vi "Inst_DAQ.vi"(8 "error in":errorcluster, 10 "All Message Queues in":T2, 11 "Prueba31 in":refnum<class "Prueba31.lvclass">) -> (0 "error out":errorcluster)   [LabVIEW 2019, in "Prueba31.lvclass"]
uses:
  Prueba31.lvclass
  QMH/Message Queue/All Message Queues.ctl
  QMH/Message Queue/Message Cluster.ctl
  Prueba31.lvclass/Prueba31.ctl
  <vilib>/DAQmx/write.llb/DAQmx Write (Analog 1D Wfm NChan NSamp).vi
  <vilib>/DAQmx/read.llb/DAQmx Read (Analog Wfm 1Chan 1Samp).vi
  <vilib>/Utility/error.llb/Error Cluster From Error Code.vi
  QMH/Message Queue/Enqueue Message (Single).vi
  <vilib>/DAQmx/create/channels.llb/DAQmx Create Channel (AO-Voltage-Basic).vi
  <vilib>/DAQmx/configure/timing.llb/DAQmx Timing (Sample Clock).vi
  <vilib>/DAQmx/miscellaneous.llb/DAQmx Fill In Error Info.vi
  <vilib>/DAQmx/create/channels.llb/DAQmx Create Channel (AI-Voltage-Basic).vi
  <vilib>/measure/matone.llb/Harmonic Distortion Analyzer 1 Chan.vi
  <vilib>/ErrorRing/Error Ring.xnode
  QMH/Message Queue/Message Queue.lvlib
  Instrumento/CNT90/CNT90.lvclass
  <vilib>/measure/NI_MAPro.lvlib
  <vilib>/measure/NI_MABase.lvlib
panel:
  in  "Output Array":T1(array[cluster])=[{"Waveform Type"=0, "Amplitude"=1.0, "Frequency"=10.0}] {"Frequency" format="%0.2p"; "Amplitude" format="%0.2p"; "Waveform Type" items=["Sine Wave", "Triangle Wave", "Square Wave", "Sawtooth Wave"]}
  out "All States":string[](array[string])
  out "Actual State":string
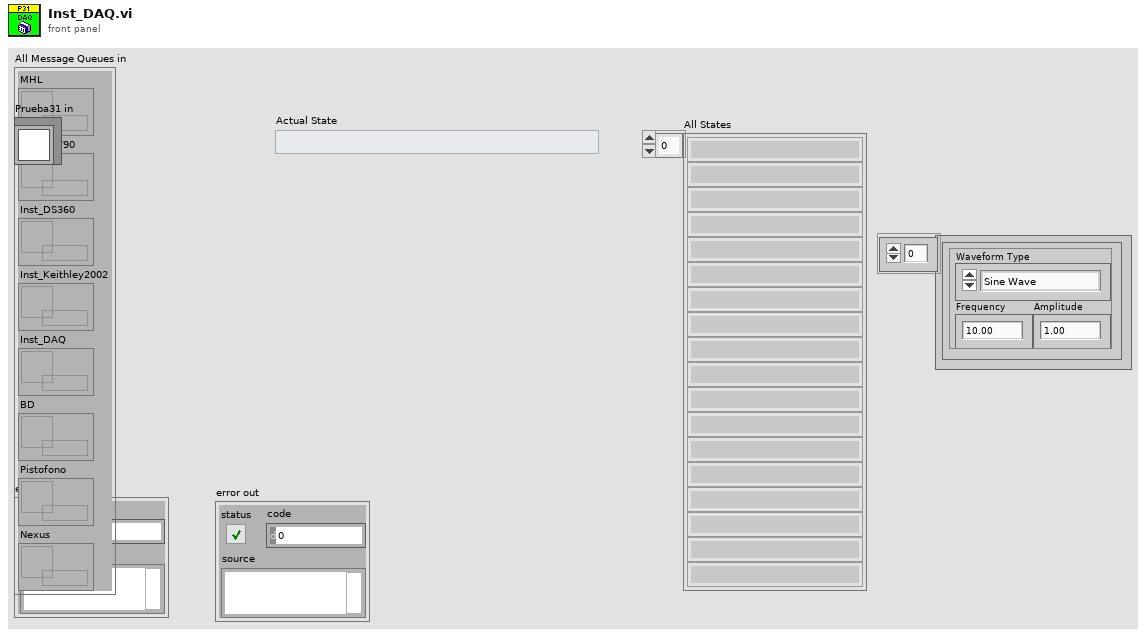
[diagram p1: front panel]
types:
  T1 = cluster{"Waveform Type":u16, "Amplitude":dbl, "Frequency":dbl}[]
  T2 = typedef "Message Queue.lvlib/All Message Queues.ctl" = cluster{"MHL":refnum<queue>, "Inst_CNT90":refnum<queue>, "Inst_DS360":refnum<queue>, "Inst_Keithley2002":refnum<queue>, "Inst_DAQ":refnum<queue>, "BD":refnum<queue>, "Pistofono":refnum<queue>, "Nexus":refnum<queue>}
  T3 = cluster{"Waveform Type":u16, "Amplitude":dbl, "Frequency":dbl}
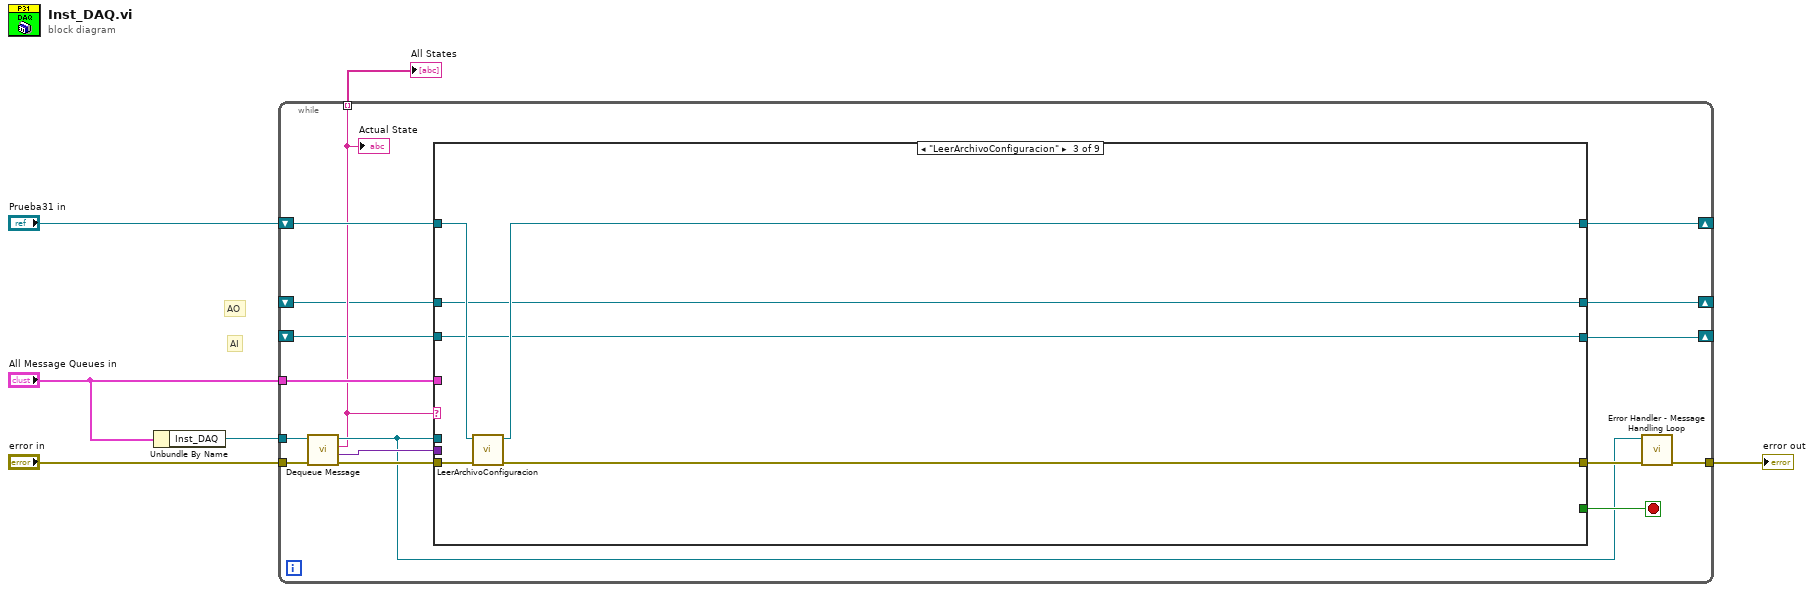
[diagram p0: block diagram]
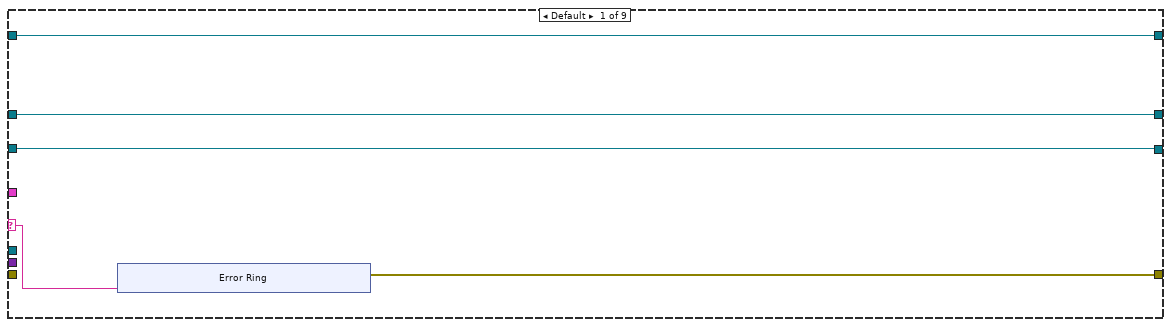
[diagram p2: hidden frame]
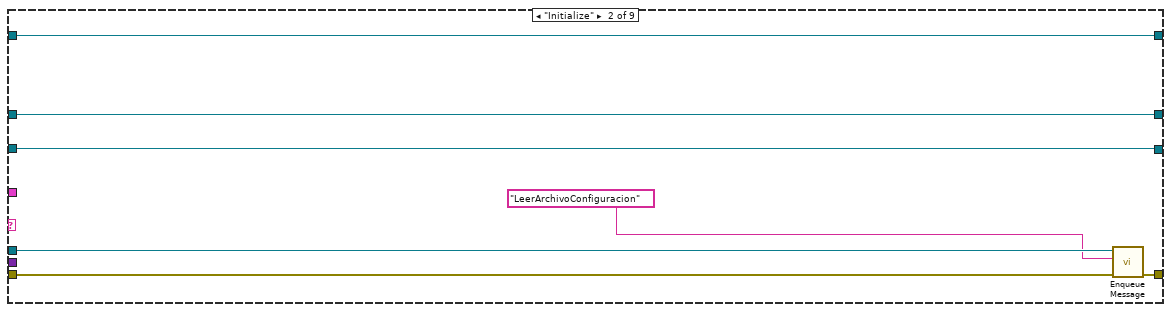
[diagram p3: hidden frame]
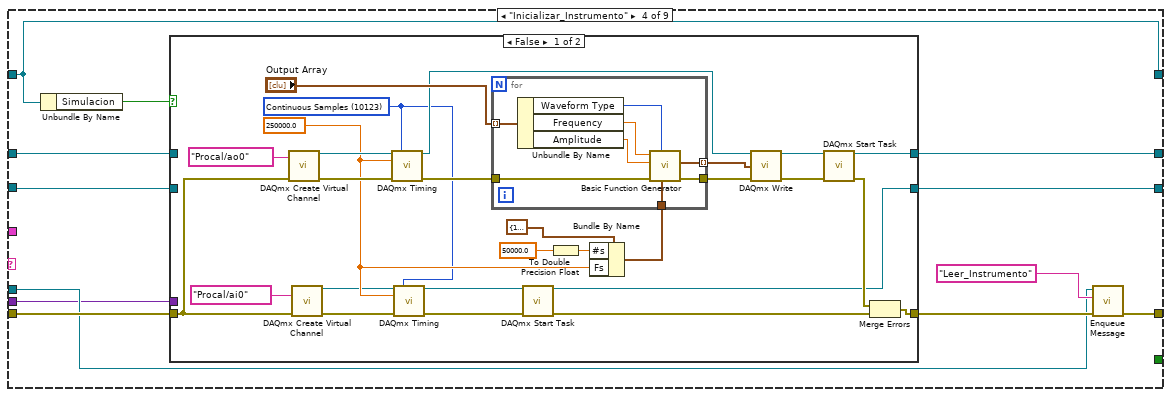
[diagram p4: hidden frame]
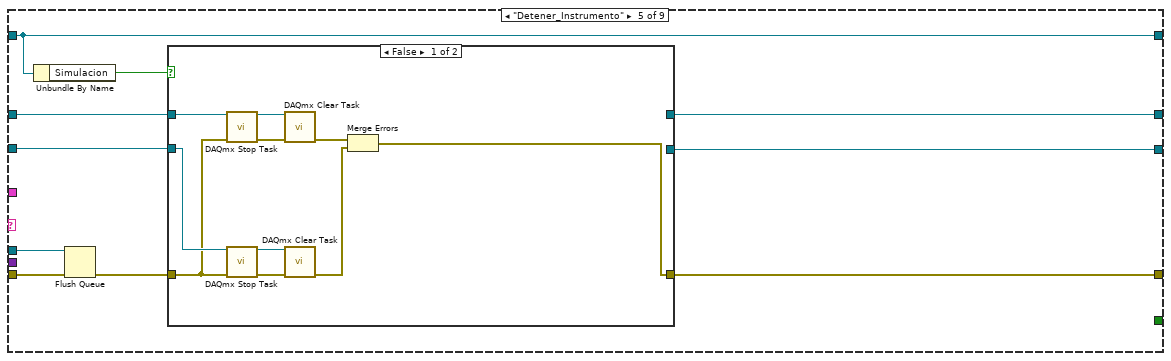
[diagram p6: hidden frame]
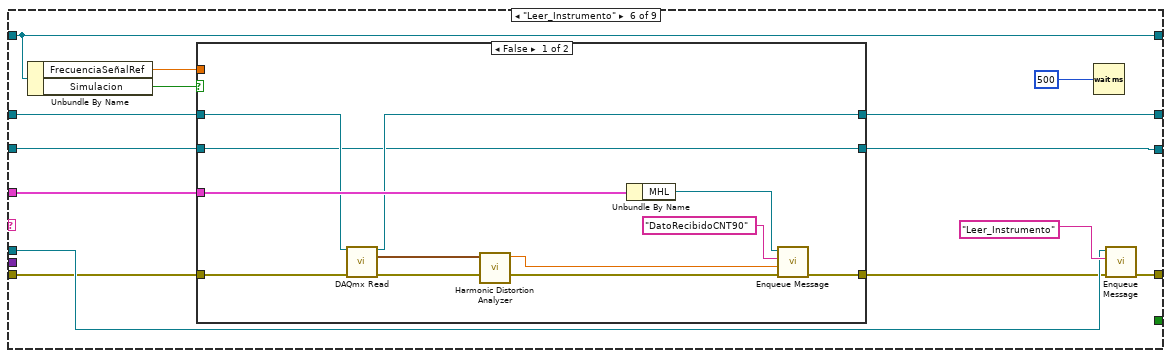
[diagram p8: hidden frame]
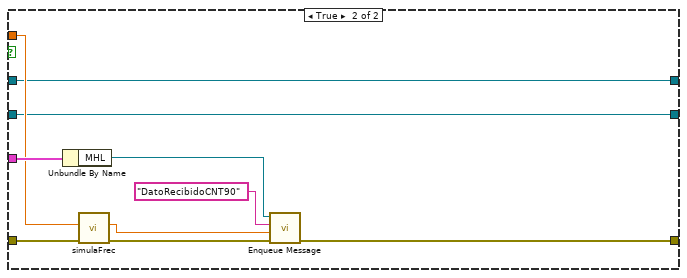
[diagram p9: hidden frame]
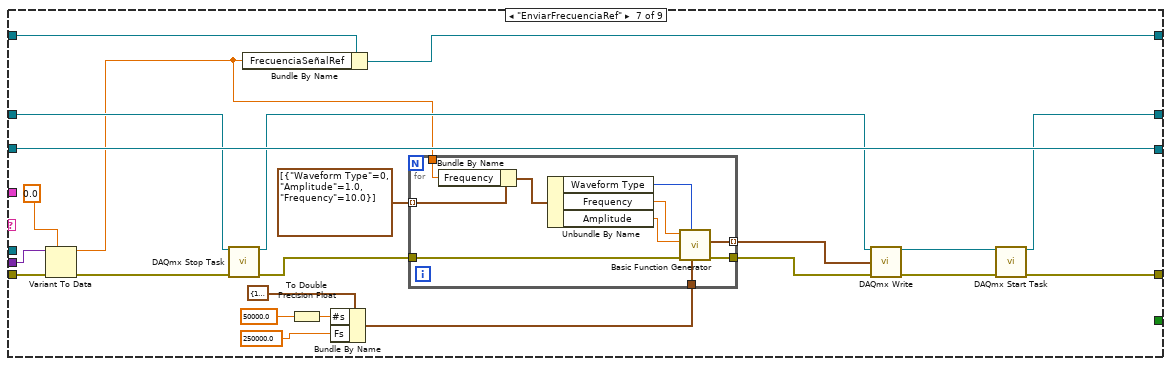
[diagram p10: hidden frame]
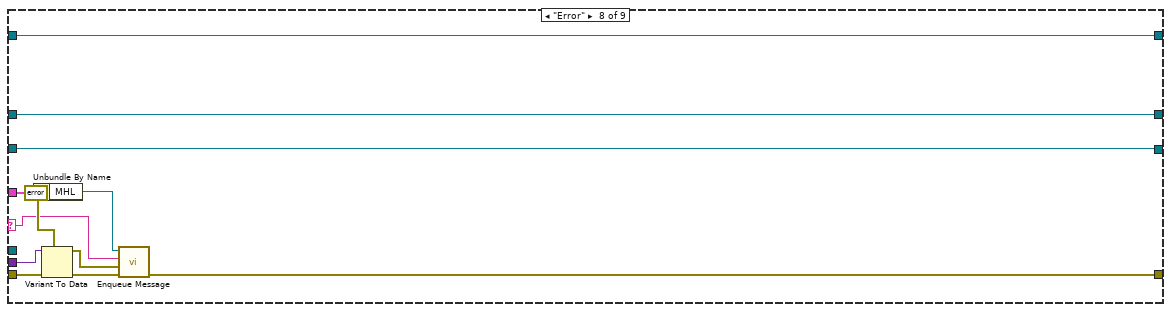
[diagram p11: hidden frame]
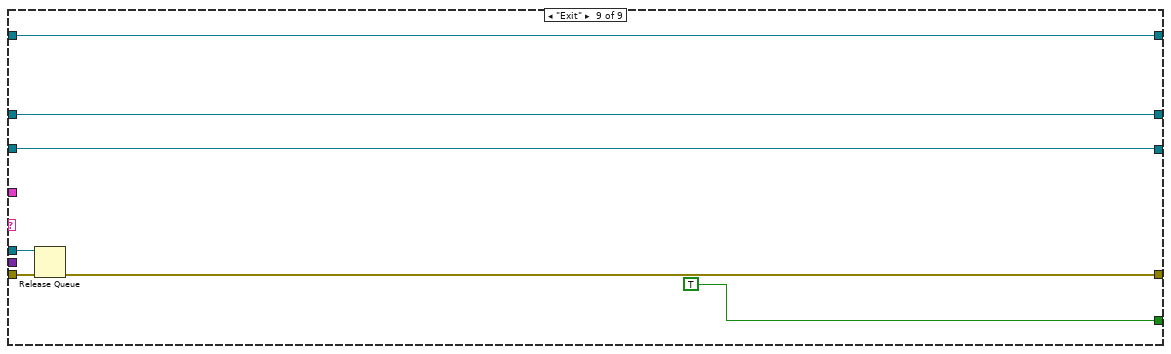
[diagram p12: hidden frame]
diagram:
  # "AI"
  # "AO"
  n1 = Unbundle By Name("All Message Queues in") -> ("Inst_DAQ"=w4:refnum<queue>)
  n2 = while {
    tunnel: "error in" -> [w22]
    tunnel: w4 -> [w21]
    tunnel: "All Message Queues in" -> [w20]
    tunnel: [w13] -> w2
    shift-right: [w16] -> _
    shift-left: "Prueba31 in" -> [w19]
    tunnel: [w11] -> w1 mode=indexing
    shift-right: [w10] -> _
    shift-left: _ -> [w8]
    shift-right: [w9] -> _
    shift-left: _ -> [w7]
    stop <- w15 stop-if-true
    n3 = call "Dequeue Message.vi"("error in (no error)"=w22, "Message Queue"=w21) -> ("error out"=w17:errorcluster, "Message Data"=w18:variant, "Message"=w11:string, "dup Message Queue"=w12:refnum<queue>)  [unwired: 6 in]
    "Actual State" <- w11
    n4 = case shown="\"LeerArchivoConfiguracion\"" w11 {
      selector: w11 -> [w27 _ _ _ _ _ _ w195 _]
      tunnel: w20 -> [_ _ _ _ _ w126 _ w194 _]
      tunnel: w19 -> [w25 w41 w45 w59 w106 w128 w174 w192 w204]
      tunnel: w12 -> [_ w38 _ w53 w102 w132 _ _ w206]
      tunnel: w18 -> [_ _ _ w52 _ _ w177 w198 _]
      tunnel: w17 -> [_ w39 w47 w58 w103 w130 w178 w199 w207]
      tunnel: [w26 w40 w44 w55 w107 w133 w158 w191 w203] -> w14
      tunnel: [w25 w41 w46 w59 w106 w128 w175 w192 w204] -> w16
      tunnel: [_ _ _ _ _ _ _ _ TRUE] -> w15
      tunnel: [w24 w36 w43 w51 w99 w123 w156 w190 w202] -> w10
      tunnel: [w23 w35 w42 w50 w98 w122 w173 w189 w201] -> w9
      tunnel: w8 -> [w24 w36 w43 w49 w100 w124 w171 w190 w202]
      tunnel: w7 -> [w23 w35 w42 w48 w101 w121 w173 w189 w201]
      frame Default {
        n5 = xnode "Error Ring"("parameter 0"=w27) -> ("error out"=w26:errorcluster)
      }
      frame "Initialize" {
        n6 = call-poly "Enqueue Message.vi"("error in (no error)"=w39, "Message"="LeerArchivoConfiguracion", "Message Queue"=w38) -> ("error out"=w40:errorcluster)  [unwired: 7 in, 1 out]
      }
      frame "LeerArchivoConfiguracion" {
        n7 = call "LeerArchivoConfiguracion.vi"("error in"=w47, "Prueba31 in"=w45) -> ("error out"=w44:errorcluster, "Prueba31 out"=w46:refnum<class "Prueba31.lvclass">)  [unwired: 8 in]
      }
      frame "Inicializar_Instrumento" {
        n8 = Unbundle By Name(w59) -> ("Simulacion"=w57:bool)
        n9 = case shown="False" w57 {
          tunnel: [w61 w97] -> w54
          tunnel: w58 -> [w84 w97]
          tunnel: w52 -> [_ _]
          tunnel: [w70 w96] -> w51
          tunnel: [w60 w95] -> w50
          tunnel: w49 -> [_ w96]
          tunnel: w48 -> [_ w95]
          frame False {
            w63 = 10123 items=["Finite Samples"=10178, "Continuous Samples"=10123, "Hardware Timed Single Point"=12522] ("sample mode")
            w67 = 250000.0 ("rate")
            n10 = call-poly <vilib>:"DAQmx Create Virtual Channel.vi"("physical channels"=tag "Procal/ao0", "error in"=w84) -> ("task out"=w83:refnum<k21>, "error out"=w82:errorcluster)  [unwired: 12 in]
            n11 = call-poly <vilib>:"DAQmx Create Virtual Channel.vi"("physical channels"=tag "Procal/ai0", "error in"=w84) -> ("task out"=w64:refnum<k21>, "error out"=w68:errorcluster)  [unwired: 12 in]
            n12 = call-poly <vilib>:"DAQmx Timing.vi"("task/channels in"=w83, "sample mode"=w63, "rate"=w67, "error in"=w82) -> ("task out"=w73:refnum<k21>, "error out"=w76:errorcluster)  [unwired: 10 in]
            n13 = call-poly <vilib>:"DAQmx Timing.vi"("task/channels in"=w64, "sample mode"=w63, "rate"=w67, "error in"=w68) -> ("task out"=w65:refnum<k21>, "error out"=w66:errorcluster)  [unwired: 10 in]
            n14 = call <vilib>:"DAQmx Start Task.vi"("task/channels in"=w65, "error in"=w66) -> ("task out"=w60:refnum<k21>, "error out"=w62:errorcluster)  [unwired: 12 in]
            n15 = To Double Precision Float(number=50000.0) -> (double precision float=w80:dbl)
            n16 = Bundle By Name(cluster=cluster{"Fs":dbl, "#s":dbl} {"Fs"=1000.0, "#s"=1000.0} ("sampling info"), "#s"=w80, "Fs"=w67) -> (w78:cluster{"Fs":dbl, "#s":dbl})
            n17 = for {
              tunnel: w78 -> [w94]
              tunnel: "Output Array" -> [w93] mode=indexing
              tunnel: [w89] -> w74 mode=indexing
              tunnel: w76 -> [w88]
              tunnel: [w87] -> w75
              n18 = Unbundle By Name(w93) -> ("Waveform Type"=w92:u16, "Frequency"=w91:dbl, "Amplitude"=w90:dbl)
              n19 = call <vilib>:"Basic Function Generator.vi"("sampling info"=w94, "signal type"=w92, "error in (no error)"=w88, "amplitude"=w90, "frequency"=w91) -> ("error out"=w87:errorcluster, "signal out"=w89:waveform(dbl))  [unwired: 4 in, 1 out]
            }
            n20 = call-poly <vilib>:"DAQmx Write.vi"("task/channels in"=w73, "data"=w74, "error in"=w75) -> ("task out"=w71:refnum<k21>, "error out"=w72:errorcluster)  [unwired: 10 in, 1 out]
            n21 = call <vilib>:"DAQmx Start Task.vi"("task/channels in"=w71, "error in"=w72) -> ("task out"=w70:refnum<k21>, "error out"=w69:errorcluster)  [unwired: 12 in]
            n22 = Merge Errors(w69, w62) -> (w61:errorcluster)
          }
          frame True {
            # "Simulacion"
          }
        }
        n23 = call-poly "Enqueue Message.vi"("error in (no error)"=w54, "Message"="Leer_Instrumento", "Message Queue"=w53) -> ("error out"=w55:errorcluster)  [unwired: 7 in, 1 out]
      }
      frame "Detener_Instrumento" {
        n24 = Unbundle By Name(w106) -> ("Simulacion"=w105:bool)
        n25 = Flush Queue(queue=w102, error in (no error)=w103) -> (error out=w104:errorcluster)  [unwired: 2 out]
        n26 = case shown="False" w105 {
          tunnel: [w108 w120] -> w107
          tunnel: w104 -> [w112 w120]
          tunnel: w101 -> [w116 w118]
          tunnel: w100 -> [w111 w119]
          tunnel: [_ w119] -> w99
          tunnel: [_ w118] -> w98
          frame False {
            n27 = call <vilib>:"DAQmx Stop Task.vi"("task/channels in"=w111, "error in"=w112) -> ("task out"=w114:refnum<k21>, "error out"=w113:errorcluster)  [unwired: 12 in]
            n28 = call <vilib>:"DAQmx Stop Task.vi"("task/channels in"=w116, "error in"=w112) -> ("task out"=w115:refnum<k21>, "error out"=w117:errorcluster)  [unwired: 12 in]
            n29 = call <vilib>:"DAQmx Clear Task.vi"("task in"=w114, "error in"=w113) -> ("error out"=w110:errorcluster)  [unwired: 13 in]
            n30 = call <vilib>:"DAQmx Clear Task.vi"("task in"=w115, "error in"=w117) -> ("error out"=w109:errorcluster)  [unwired: 13 in]
            n31 = Merge Errors(w110, w109) -> (w108:errorcluster)
          }
          frame True {
          }
        }
      }
      frame "Leer_Instrumento" {
        n32 = Unbundle By Name(w128) -> ("FrecuenciaSeñalRef"=w125:dbl, "Simulacion"=w127:bool)
        n33 = case shown="False" w127 {
          tunnel: [w144 w154] -> w129
          tunnel: w130 -> [w139 w151]
          tunnel: w126 -> [w143 w153]
          tunnel: w125 -> [_ w148]
          tunnel: w124 -> [w137 w147]
          tunnel: [w136 w147] -> w123
          tunnel: [w135 w146] -> w122
          tunnel: w121 -> [w135 w146]
          frame False {
            n34 = call-poly <vilib>:"DAQmx Read.vi"("task/channels in"=w137, "error in"=w139) -> ("task out"=w136:refnum<k21>, "data"=w141:waveform(dbl), "error out"=w140:errorcluster)  [unwired: 11 in]
            n35 = call-poly <vilib>:"Harmonic Distortion Analyzer.vi"("signal in"=w141) -> ("detected fundamental frequency"=w138:dbl)  [unwired: 5 in, 5 out]
            n36 = Unbundle By Name(w143) -> ("MHL"=w142:refnum<queue>)
            n37 = call-poly "Enqueue Message.vi"("error in (no error)"=w140, "Message Data"=w138, "Message"="DatoRecibidoCNT90", "Message Queue"=w142) -> ("error out"=w144:errorcluster)  [unwired: 6 in, 1 out]
          }
          frame True {
            n38 = Unbundle By Name(w153) -> ("MHL"=w152:refnum<queue>)
            n39 = call "simulaFrec.vi"("error in (no error)"=w151, "frec in"=w148) -> ("error out"=w150:errorcluster, "frec out"=w149:dbl)  [unwired: 7 in, 1 out]
            n40 = call-poly "Enqueue Message.vi"("error in (no error)"=w150, "Message Data"=w149, "Message"="DatoRecibidoCNT90", "Message Queue"=w152) -> ("error out"=w154:errorcluster)  [unwired: 6 in, 1 out]
          }
        }
        n41 = Wait (ms)(milliseconds to wait=u32 500) -> ()  [unwired: 1 out]
        n42 = call-poly "Enqueue Message.vi"("error in (no error)"=w129, "Message"="Leer_Instrumento", "Message Queue"=w132) -> ("error out"=w133:errorcluster)  [unwired: 7 in, 1 out]
      }
      frame "EnviarFrecuenciaRef" {
        n43 = Variant To Data(error in=w178, type=0.0, Variant=w177) -> (data=w161:dbl, error out=w172:errorcluster)
        n44 = call <vilib>:"DAQmx Stop Task.vi"("task/channels in"=w171, "error in"=w172) -> ("task out"=w163:refnum<k21>, "error out"=w165:errorcluster)  [unwired: 12 in]
        n45 = Bundle By Name(cluster=w174, "FrecuenciaSeñalRef"=w161) -> (w175:refnum<class "Prueba31.lvclass">)
        n46 = To Double Precision Float(number=50000.0) -> (double precision float=w169:dbl)
        n47 = Bundle By Name(cluster=cluster{"Fs":dbl, "#s":dbl} {"Fs"=1000.0, "#s"=1000.0} ("sampling info"), "#s"=w169, "Fs"=250000.0 ("rate")) -> (w170:cluster{"Fs":dbl, "#s":dbl})
        n48 = for {
          tunnel: w170 -> [w188]
          tunnel: T1 [{"Waveform Type"=0, "Amplitude"=1.0, "Frequency"=10.0}] ("Output Array 2") -> [w180] mode=indexing
          tunnel: [w184] -> w160 mode=indexing
          tunnel: w165 -> [w183]
          tunnel: [w182] -> w164
          tunnel: w161 -> [w179]
          n49 = Bundle By Name(cluster=w180, "Frequency"=w179) -> (w181:T3)
          n50 = Unbundle By Name(w181) -> ("Waveform Type"=w187:u16, "Frequency"=w186:dbl, "Amplitude"=w185:dbl)
          n51 = call <vilib>:"Basic Function Generator.vi"("sampling info"=w188, "signal type"=w187, "error in (no error)"=w183, "amplitude"=w185, "frequency"=w186) -> ("error out"=w182:errorcluster, "signal out"=w184:waveform(dbl))  [unwired: 4 in, 1 out]
        }
        n52 = call-poly <vilib>:"DAQmx Write.vi"("task/channels in"=w163, "data"=w160, "error in"=w164) -> ("task out"=w157:refnum<k21>, "error out"=w159:errorcluster)  [unwired: 10 in, 1 out]
        n53 = call <vilib>:"DAQmx Start Task.vi"("task/channels in"=w157, "error in"=w159) -> ("task out"=w156:refnum<k21>, "error out"=w158:errorcluster)  [unwired: 12 in]
      }
      frame "Error" {
        n54 = Unbundle By Name(w194) -> ("MHL"=w193:refnum<queue>)
        n55 = Variant To Data(error in=w199, type=errorcluster {"status"=FALSE, "code"=0, "source"=""} ("error constant"), Variant=w198) -> (data=w196:errorcluster, error out=w197:errorcluster)
        n56 = call-poly "Enqueue Message.vi"("error in (no error)"=w197, "Message Data"=w196, "Message"=w195, "Message Queue"=w193) -> ("error out"=w191:errorcluster)  [unwired: 6 in, 1 out]
      }
      frame "Exit" {
        n57 = Release Queue(queue=w206, error in (no error)=w207) -> (error out=w203:errorcluster)  [unwired: 1 in, 2 out]
      }
    }
    n58 = call "Error Handler - Message Handling Loop.vi"("error in (no error)"=w14, "Message Queue"=w12) -> ("dup error in"=w13:errorcluster)  [unwired: 8 in, 1 out]
  }
  "error out" <- w2
  "All States" <- w1
